vi "Instr panel replacement.vi"() -> ()   [LabVIEW 2017]
uses:
  Instruments/Spectrometer Triax 550/Spectrometer Triax 550.lvclass
panel:
  out "error out":errorcluster
  in  "error in (no error)":errorcluster
  in  "JY Triax spectrometer control":bool
  out "Array of statuses (newest on top)":string[](array[string])
  in  "stop":bool
  in  "JY Triax spectrometer status":bool
  out "special JY Triax status":string
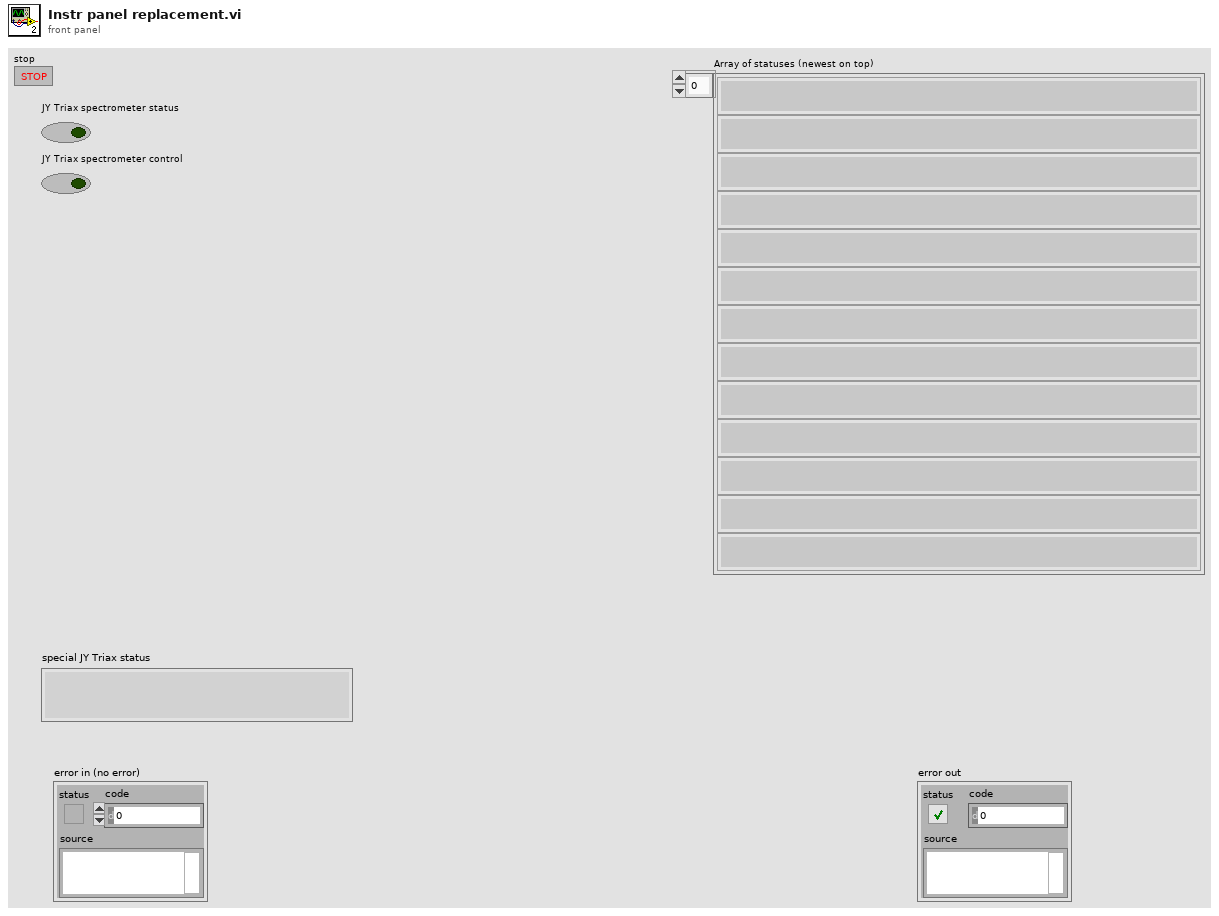
[diagram p1: front panel]
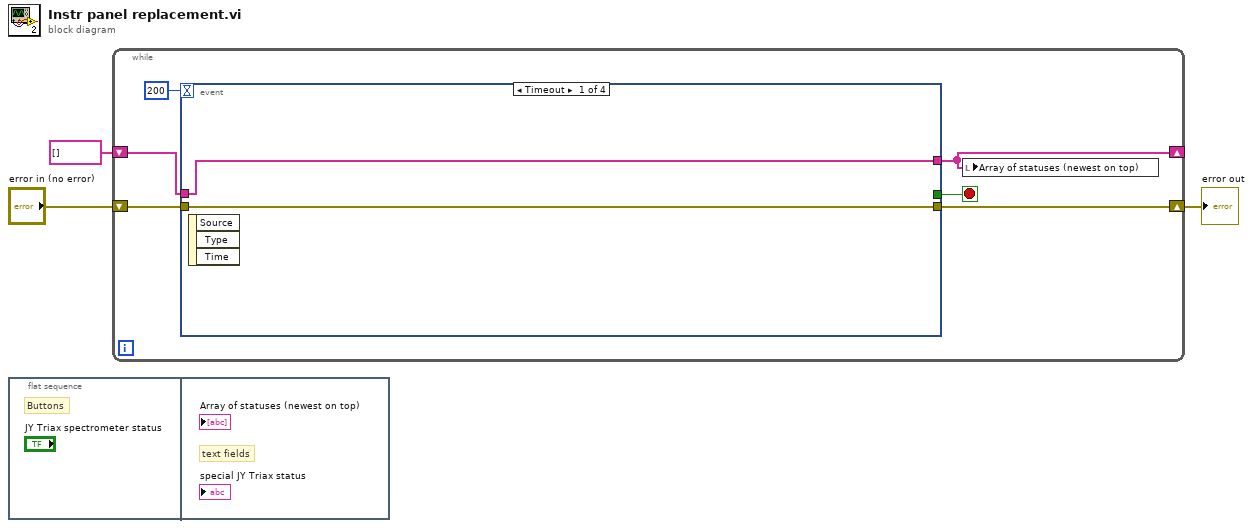
[diagram p0: block diagram]
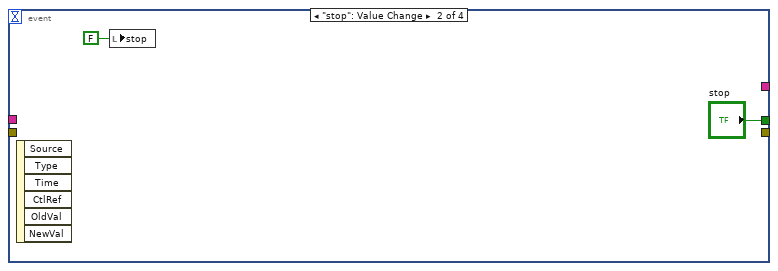
[diagram p2: hidden frame]
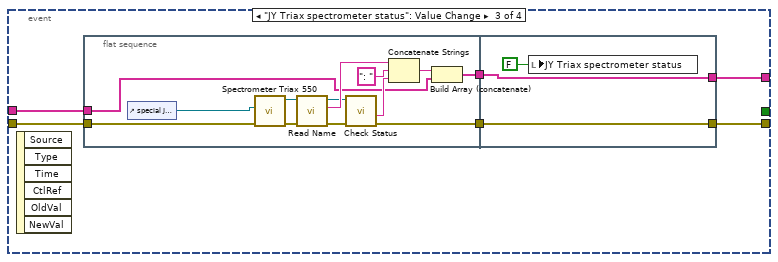
[diagram p3: hidden frame]
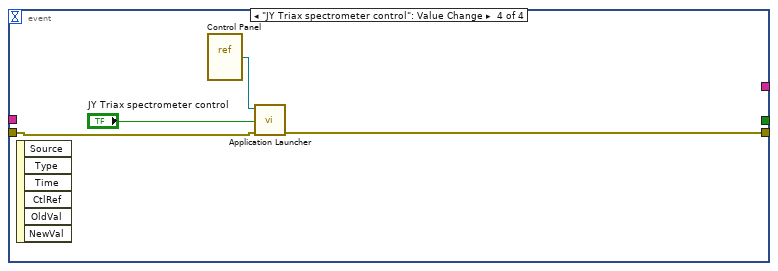
[diagram p4: hidden frame]
diagram:
  n1 = flat-sequence {
    frame #0 {
      # "Buttons"
    }
    frame #1 {
      # "text fields"
    }
  }
  n2 = while {
    shift-right: [w7] -> _
    shift-left: string[] [] -> [w8]
    shift-right: [w5] -> w1
    shift-left: "error in (no error)" -> [w6]
    stop <- w9 stop-if-true
    n3 = event shown="[0] Timeout" {
      selector: _ -> [_ _ _ _]
      dyn-events: _ -> [_ _ _ _]
      timeout: 200 -> [_ _ _ _]
      tunnel: [_ "stop" _ _] -> w9
      tunnel: w8 -> [w11 _ w19 _]
      tunnel: [w11 _ w18 _] -> w7
      tunnel: w6 -> [w10 _ w16 w39]
      tunnel: [w10 _ w15 w38] -> w5
      event Timeout {
        n4 = event-data() -> ()  [unwired: 1 in, 3 out]
      }
      event "stop": Value Change {
        n5 = event-data() -> ()  [unwired: 1 in, 6 out]
        n6 = local write "stop"(FALSE ("stop")) -> ()
      }
      event "JY Triax spectrometer status": Value Change {
        n7 = event-data() -> ()  [unwired: 1 in, 6 out]
        n8 = flat-sequence {
          tunnel: w19 -> [w20]
          tunnel: [w24] -> w17
          tunnel: w16 -> [w23]
          tunnel: [w22] -> w14
          tunnel: [w34] -> w18
          tunnel: w17 -> [w34]
          tunnel: [w33] -> w15
          tunnel: w14 -> [w33]
          frame #0 {
            n9 = control-ref of="special JY Triax status"() -> (w32:refnum<vi>)
            n10 = call "Spectrometer Triax 550.vi"("error in (no error)"=w23, "Ref to a Status Box"=w32) -> ("error out"=w25:errorcluster, "Spectrometer Triax 550 out"=w31:refnum<class "Spectrometer Triax 550.lvclass">)  [unwired: 1 in, 7 out]
            n11 = call-dynamic "Read Name.vi"("error in (no error)"=w25, "Spectrometer Triax 550.lvclass in"=w31) -> ("error out"=w26:errorcluster, "Name"=w29:string, "Spectrometer Triax 550.lvclass out"=w27:refnum<class "Spectrometer Triax 550.lvclass">)  [unwired: 7 out]
            n12 = call-dynamic "Check Status.vi"("error in (no error)"=w26, "Spectrometer Triax 550 in"=w27) -> ("error out"=w22:errorcluster, "Status"=w28:string)  [unwired: 6 in, 2 out]
            n13 = Concatenate Strings(w29, ": " ("string"), w28) -> (w21:string)
            n14 = Build Array (concatenate)(w21, w20) -> (w24:string[])
          }
          frame #1 {
            n15 = local write "JY Triax spectrometer status"(FALSE ("JY Triax spectrometer")) -> ()
          }
        }
      }
      event "JY Triax spectrometer control": Value Change {
        n16 = event-data() -> ()  [unwired: 1 in, 6 out]
        n17 = vi-ref "Control Panel.vi"() -> (w37:refnum<vi>)
        n18 = call "Application Launcher.vi"("error in (no error)"=w39, "Toggle?"="JY Triax spectrometer control", "VI reference"=w37) -> ("error out"=w38:errorcluster)  [unwired: 1 in, 7 out]
      }
    }
    n19 = local write "Array of statuses (newest on top)"(w7) -> ()
  }
  "error out" <- w1
